vi "Bytes to Words.vi"(11 "bytes":i32) -> (3 "U16 words":u16)   [LabVIEW 2020, in "Ballard MIL-STD-1553 Engine.lvlib" / "Implementation.lvlib" / "Logging Execution Unit.lvclass"]
uses:
  Logging Execution Unit.lvclass
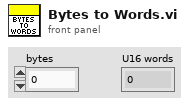
[diagram p1: front panel]
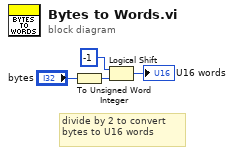
[diagram p0: block diagram]
diagram:
  # "divide by 2 to convert bytes to U16 words"
  n1 = To Unsigned Word Integer(number="bytes") -> (unsigned 16bit integer=w1:u16)
  n2 = Logical Shift(y=i16 -1, x=w1) -> (x << y=→"U16 words":u16)
